vi "ManualControlGlobal.vi"() -> ()   [LabVIEW 2013]
panel:
  in  "TTspeed":dbl
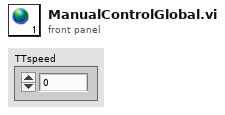
[diagram p1: front panel]
diagram:
